vi "Analytics.vi"(8 "error in":errorcluster, 10 "Cluster Of Graphs":T1, 11 "User Event References":T2) -> (0 "error out":errorcluster)   [LabVIEW 2015]
uses:
  TypeDef/User Event References.ctl
  TypeDef/GetData Cluster.ctl
  TypeDef/ResultUpdate Cluster.ctl
  TypeDef/Initialize_Cluster.ctl
  TypeDef/OverWrite JSON Cluster.ctl
  TypeDef/GraphReff.ctl
  TypeDef/UE Reference For Plot.ctl
  TypeDef/Plot Cluster.ctl
types:
  T1 = typedef "GraphReff.ctl" = cluster{"HistgramGraph-reff":refnum<vi>[], "BarGraph-reff":refnum<vi>[], "PieGraph-reff":refnum<vi>[], "Lable-reff":refnum<vi>[], "TrendGraph-reff":refnum<vi>[], "CpCpkTable":refnum<vi>}
  T2 = typedef "User Event References.ctl" = cluster{"Measurement":refnum<user-event>, "Stop_M":refnum<user-event>, "Exit_M":refnum<user-event>, "Analytics":refnum<user-event>, "Back":refnum<user-event>, "Getdata":refnum<user-event>, "ResultUpdate":refnum<user-event>, "Pause_M":refnum<user-event>, "Stop_Analytics":refnum<user-event>, "Exit_Analytics ":refnum<user-event>, "Measurement_M":refnum<user-event>, "Pause_Analytics":refnum<user-event>, "Initialization":refnum<user-event>, "Feedback_Pause":refnum<user-event>, "Feedback_Stop":refnum<user-event>, "Feedback_Exit":refnum<user-event>, "Override JSON":refnum<user-event>}
  T3 = typedef "Plot Cluster.ctl" = cluster{"Reduced 2D":dbl[][], "Start Index":i32, "MeasurementData":cluster{"MeasurementID":i32, "MeasureEnable":bool, "MeasurementPass":bool, "LimitSets":cluster{"LimitSetId":i32, "Limits":dbl[]}[]}[], "No Of New Termnals":i32, "Top/Bottom":bool, "Values Inserted":i32, "PlotParameters":cluster{"Trend":cluster{"TrendID":i32, "PlotEnable":bool, "PlotTitle":string, "PlotCaptionFont":cluster{"FontName":string, "FontSize":i32, "IsBold":bool, "IsItalic":bool, "IsUnderline":bool, "IsStrikeout":bool, "FontColor":string}, "XLabel":string, "XLabelFont":cluster{"FontName":string, "FontSize":i32, "IsBold":bool, "IsItalic":bool, "IsUnderline":bool, "IsStrikeout":bool, "FontColor":string}, "SamplesToDisplay":i32, "Channels":cluster{"Label":string, "YLabelFont":cluster{"FontName":string, "FontSize":i32, "IsBold":bool, "IsItalic":bool, "IsUnderline":bool, "IsStrikeout":bool, "FontColor":string}, "MeasurementID":i32, "PlotColor":string, "PointShape":string, "ShowOnGraph":bool}[]}[], "Histogram":cluster{"HistogramID":i32, "PlotEnable":bool, "PlotTitle":string, "PlotLabelFont":cluster{"FontName":string, "FontSize":i32, "IsBold":bool, "IsItalic":bool, "IsUnderline":bool, "IsStrikeout":bool, "FontColor":string}, "XLabel":string, "XLabelFont":cluster{"FontName":string, "FontSize":i32, "IsBold":bool, "IsItalic":bool, "IsUnderline":bool, "IsStrikeout":bool, "FontColor":string}, "YLabel":string, "YLabelFont":cluster{"FontName":string, "FontSize":i32, "IsBold":bool, "IsItalic":bool, "IsUnderline":bool, "IsStrikeout":bool, "FontColor":string}, "MeasurementID":i32, "PlotColor":string, "SamplesToDisplay":i32}[], "BarPlot":cluster{"BarPlotID":i32, "BarValuesID":i32, "PlotEnable":bool, "PlotLabel":string, "PlotLabelFont":cluster{"FontName":string, "FontSize":i32, "IsBold":bool, "IsItalic":bool, "IsUnderline":bool, "IsStrikeout":bool, "FontColor":string}, "XLabel":string, "XLabelFont":cluster{"FontName":string, "FontSize":i32, "IsBold":bool, "IsItalic":bool, "IsUnderline":bool, "IsStrikeout":bool, "FontColor":string}, "YLabel":string, "YLabelFont":cluster{"FontName":string, "FontSize":i32, "IsBold":bool, "IsItalic":bool, "IsUnderline":bool, "IsStrikeout":bool, "FontColor":string}, "Sectors":string[]}[], "PieChart":cluster{"PieChartID":i32, "PieChartValueID":i32, "PlotEnable":bool, "PlotLabel":string, "PlotLabelFont":cluster{"FontName":string, "FontSize":i32, "IsBold":bool, "IsItalic":bool, "IsUnderline":bool, "IsStrikeout":bool, "FontColor":string}, "Sectors":string[]}[]}, "Re-Initialised":bool, "Statistical params":string[][], "MeasurementData_IndexValues":cluster{"Measurement-ID":i32[], "Measurement-Enable":bool[], "LSL":dbl[], "USL":dbl[]}}
  T4 = typedef "UE Reference For Plot.ctl" = cluster{"Stop_Plot":refnum<user-event>, "Exit_PLot":refnum<user-event>, "Plot":refnum<user-event>, "CpCpkData":refnum<user-event>}
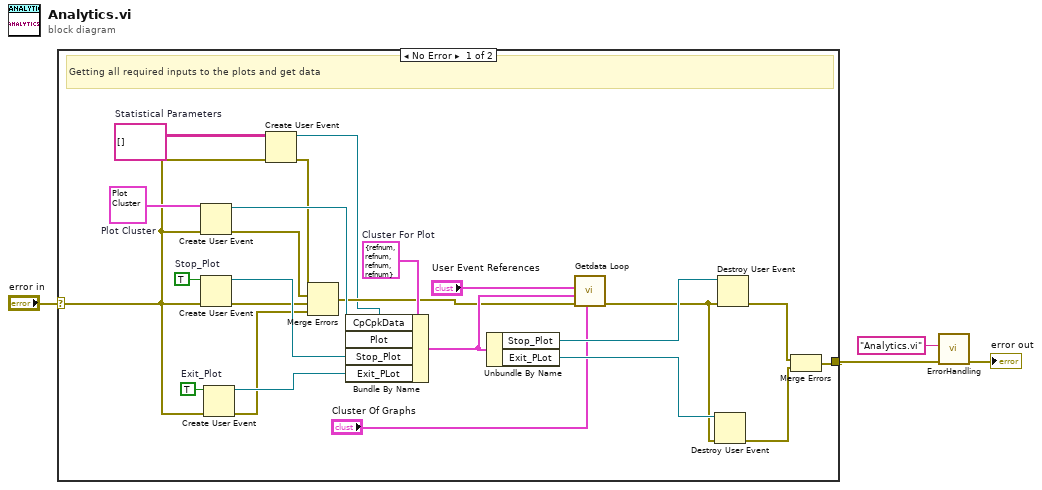
[diagram p0: block diagram]
diagram:
  n1 = case shown="No Error" "error in" {
    selector: "error in" -> [w7 w29]
    tunnel: [w15 w29] -> w3
    frame No Error {
      w11 = string[][] []  # Statistical Parameters
      w14 = T3 {"Reduced 2D"=[], "Start Index"=0, "MeasurementData"=[], "No Of New Termnals"=0, "Top/Bottom"=FALSE, "Values Inserted"=0, "PlotParameters"={"Trend"=[], "Histogram"=[], "BarPlot"=[], "PieChart"=[]}, "Re-Initialised"=FALSE, "Statistical params"=[], "MeasurementData_IndexValues"={"Measurement-ID"=[], "Measurement-Enable"=[], "LSL"=[], "USL"=[]}}  # Plot Cluster
      w24 = T4 {"Stop_Plot"=refnum, "Exit_PLot"=refnum, "Plot"=refnum, "CpCpkData"=refnum}  # Cluster For Plot
      w27 = TRUE  # Exit_Plot
      w28 = TRUE  # Stop_Plot
      # "Getting all required inputs to the plots and get data"
      n2 = Create User Event(user event datatype=w14, error in=w7) -> (user event=w13:refnum<user-event>, error out=w12:errorcluster)
      n3 = Create User Event(user event datatype=w28, error in=w7) -> (user event=w26:refnum<user-event>, error out=w23:errorcluster)
      n4 = Create User Event(user event datatype=w27, error in=w7) -> (user event=w25:refnum<user-event>, error out=w22:errorcluster)
      n5 = Create User Event(user event datatype=w11, error in=w7) -> (user event=w9:refnum<user-event>, error out=w8:errorcluster)
      n6 = Merge Errors(w8, w12, w23, w22) -> (w10:errorcluster)
      n7 = Bundle By Name(cluster=w24, "CpCpkData"=w9, "Plot"=w13, "Stop_Plot"=w26, "Exit_PLot"=w25) -> (w17:T4)
      n8 = Unbundle By Name(w17) -> ("Stop_Plot"=w21:refnum<user-event>, "Exit_PLot"=w20:refnum<user-event>)
      n9 = call "Getdata Loop.vi"("Cluster Of Graphs"="Cluster Of Graphs", "error in"=w10, "Reference For PLot"=w17, "User Event References"="User Event References") -> ("error out"=w5:errorcluster)  [unwired: 7 in]
      n10 = Destroy User Event(user event=w20, error in=w5) -> (error out=w18:errorcluster)
      n11 = Destroy User Event(user event=w21, error in=w5) -> (error out=w19:errorcluster)
      n12 = Merge Errors(w19, w18) -> (w15:errorcluster)
    }
    frame Error {
    }
  }
  n13 = call "ErrorHandling.vi"("error in (no error)"=w3, "Vi-name"="Analytics.vi") -> ("error out"=→"error out":errorcluster)  [unwired: 9 in]
